vi "AuMT8852B EDR Sensitivity Extended Results.vi"(5 "Stage":T2(ring), 8 "error in (no error)":errorcluster, 11 "VISA session":refnum<visa-resource-name>) -> (0 "error out":errorcluster, 2 "error code":i32, 3 "VISA session out":refnum<visa-resource-name>, 4 "Results":T1 {"3MBs Overall BER" format="%.2e"; "2MBs Overall BER" format="%.2e"})   [LabVIEW 2017]
doc: "Anritsu MT8852B Bluetooth Tester\n\nReturns the results of the EDR Sensitivity test.\n\nINPUTS\nStage - results of the individual hopping stages of the test.\n\nOUTPUTS\nResults - measurements made during the test."
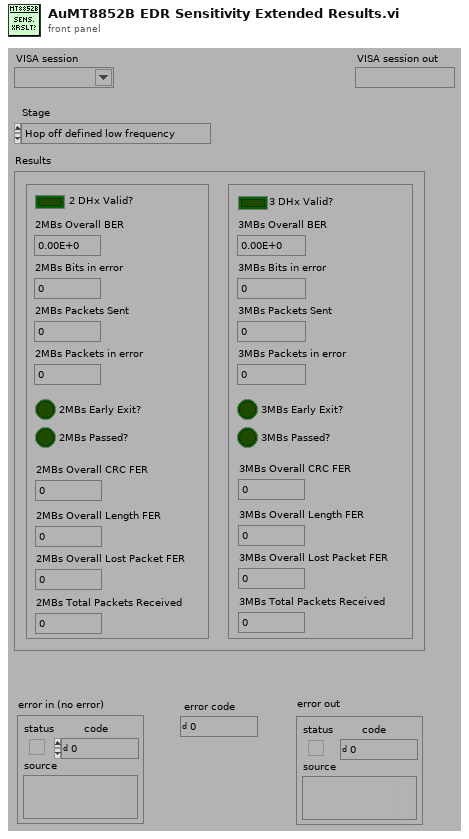
[diagram p1: front panel]
types:
  T1 = cluster{"2 DHx Valid?":bool, "2MBs Overall BER":dbl, "2MBs Bits in error":u32, "2MBs Packets Sent":u32, "2MBs Early Exit?":bool, "2MBs Packets in error":u32, "3 DHx Valid?":bool, "3MBs Overall BER":dbl, "3MBs Bits in error":u32, "3MBs Packets Sent":u32, "3MBs Early Exit?":bool, "3MBs Packets in error":u32, "2MBs Overall CRC FER":u32, "2MBs Overall Length FER":u32, "2MBs Overall Lost Packet FER":u32, "3MBs Overall CRC FER":u32, "3MBs Overall Length FER":u32, "3MBs Overall Lost Packet FER":u32, "2MBs Total Packets Received":u32, "3MBs Total Packets Received":u32, "2MBs Passed?":bool, "3MBs Passed?":bool}
  T2 = enum16{"Hop off defined low frequency", "Hop off defined medium frequency", "Hop off defined high frequency", "Hop on any channels"}
  T3 = enum16{"Simulate", "Range check", "Cache", "Query instrument status"}
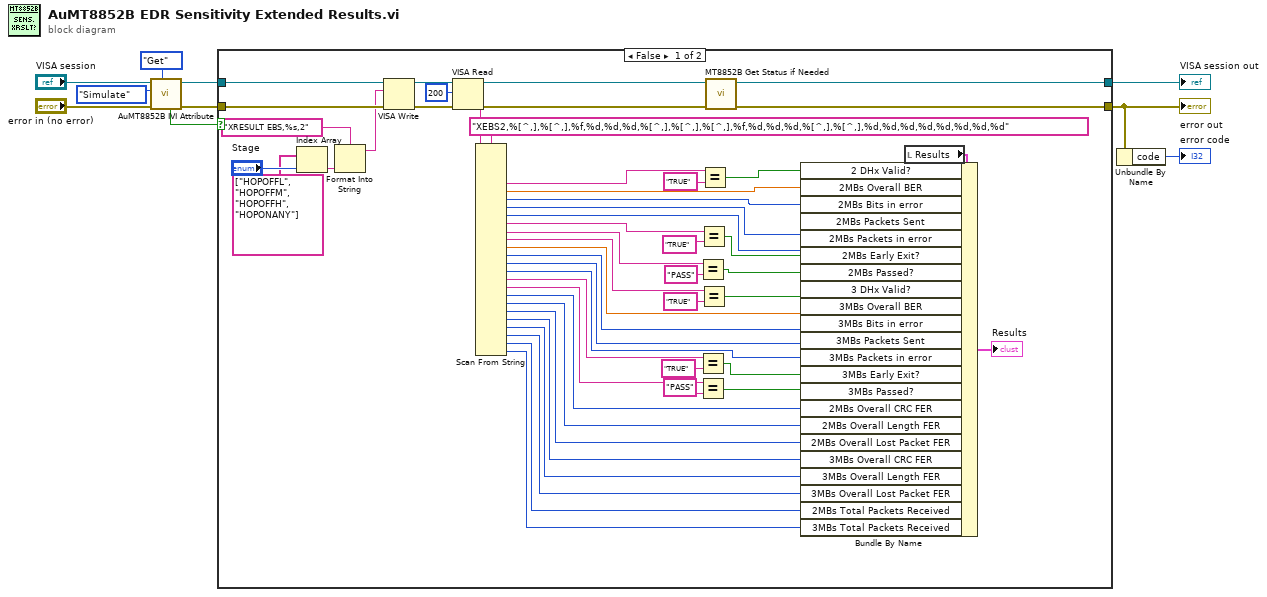
[diagram p0: block diagram]
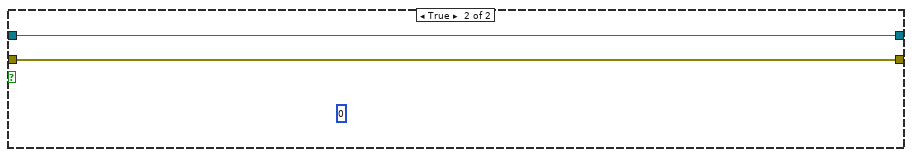
[diagram p2: hidden frame]
diagram:
  n1 = call <instrlib>:"AuMT8852B IVI Attribute.vi"("Set/Get (Set)"=enum16{"Set", "Get"}."Get", "error in (no error)"="error in (no error)", "Flag (Simulate)"=T3."Simulate", "VISA session"="VISA session") -> ("error out"=w7:errorcluster, "VISA session out"=w9:refnum<visa-resource-name>, "Value out"=w3:bool)  [unwired: 5 in]
  n2 = case shown="False" w3 {
    tunnel: [w56 w64] -> w10
    tunnel: [w55 w63] -> w1
    tunnel: w9 -> [w62 w64]
    tunnel: w7 -> [w61 w63]
    frame False {
      n3 = Index Array(array=string[] ["HOPOFFL", "HOPOFFM", "HOPOFFH", "HOPONANY"], index="Stage") -> (element=w47:string)
      n4 = Format Into String(format string="XRESULT EBS,%s,2" ("write buffer (\"\")"), w47) -> (resulting string=w44:string)  [unwired: 2 in, 1 out]
      n5 = VISA Write(VISA resource name=w62, write buffer=w44, error in (no error)=w61) -> (VISA resource name out=w60:refnum<visa-resource-name>, error out=w59:errorcluster)  [unwired: 1 out]
      n6 = VISA Read(VISA resource name=w60, byte count=u32 200 ("byte count (0)"), error in (no error)=w59) -> (VISA resource name out=w54:refnum<visa-resource-name>, read buffer=w42:string, error out=w53:errorcluster)  [unwired: 1 out]
      n7 = Scan From String(format string="XEBS2,%[^,],%[^,],%f,%d,%d,%d,%[^,],%[^,],%[^,],%f,%d,%d,%d,%[^,],%[^,],%d,%d,%d,%d,%d,%d,%d,%d" ("Format String"), input string=w42) -> (output 2=w41:string, output 3=w29:dbl, output 4=w16:i32, output 5=w31:i32, output 6=w30:i32, output 7=w23:string, output 8=w40:string, output 9=w24:string, output 10=w32:dbl, output 11=w33:i32, output 12=w34:i32, output 13=w35:i32, output 14=w36:string, output 15=w39:string, output 16=w22:i32, output 17=w21:i32, output 18=w20:i32, output 19=w15:i32, output 20=w14:i32, output 21=w13:i32, output 22=w12:i32, output 23=w11:i32)  [unwired: 26 in, 3 out]
      n8 = Equal?(x=w40, y="PASS") -> (x = y?=w27:bool)
      n9 = Equal?(x=w36, y="TRUE") -> (x = y?=w17:bool)
      n10 = Equal?(x=w39, y="PASS") -> (x = y?=w38:bool)
      n11 = Equal?(x=w23, y="TRUE") -> (x = y?=w28:bool)
      n12 = Equal?(x=w24, y="TRUE") -> (x = y?=w25:bool)
      n13 = Equal?(x=w41, y="TRUE") -> (x = y?=w52:bool)
      n14 = call <instrlib>:"MT8852B Get Status if Needed.vi"("error in (no error)"=w53, "VISA session"=w54) -> ("error out"=w55:errorcluster, "VISA session out"=w56:refnum<visa-resource-name>)  [unwired: 8 in]
      n15 = local read "Results"() -> (w19:T1)
      n16 = Bundle By Name(cluster=w19, "2 DHx Valid?"=w52, "2MBs Overall BER"=w29, "2MBs Bits in error"=w16, "2MBs Packets Sent"=w31, "2MBs Packets in error"=w30, "2MBs Early Exit?"=w28, "2MBs Passed?"=w27, "3 DHx Valid?"=w25, "3MBs Overall BER"=w32, "3MBs Bits in error"=w33, "3MBs Packets Sent"=w34, "3MBs Packets in error"=w35, "3MBs Early Exit?"=w17, "3MBs Passed?"=w38, "2MBs Overall CRC FER"=w22, "2MBs Overall Length FER"=w21, "2MBs Overall Lost Packet FER"=w20, "3MBs Overall CRC FER"=w15, "3MBs Overall Length FER"=w14, "3MBs Overall Lost Packet FER"=w13, "2MBs Total Packets Received"=w12, "3MBs Total Packets Received"=w11) -> (→"Results":T1)
    }
    frame True {
      (unwired) u8 0
    }
  }
  "error out" <- w1
  "VISA session out" <- w10
  n17 = Unbundle By Name(w1) -> ("code"=→"error code":i32)
